vi "Camera Get connected Cameras.vi"() -> (1 "Product":string[](array[string]), 3 "Camera List":string[](array[string]))   [LabVIEW 2025]
uses:
  <vilib>/vision/driver/NI_Vision_Acquisition_Software.lvlib
panel:
  out "Camera Information Array 2":T1(array[cluster]) {"BusType" format="%x"; "SerialNumberLow" format="%.0x"; "SerialNumberHigh" format="%.0x"}
  out "Camera Information Array":T1(array[cluster]) {"BusType" format="%x"; "SerialNumberLow" format="%.0x"; "SerialNumberHigh" format="%.0x"}
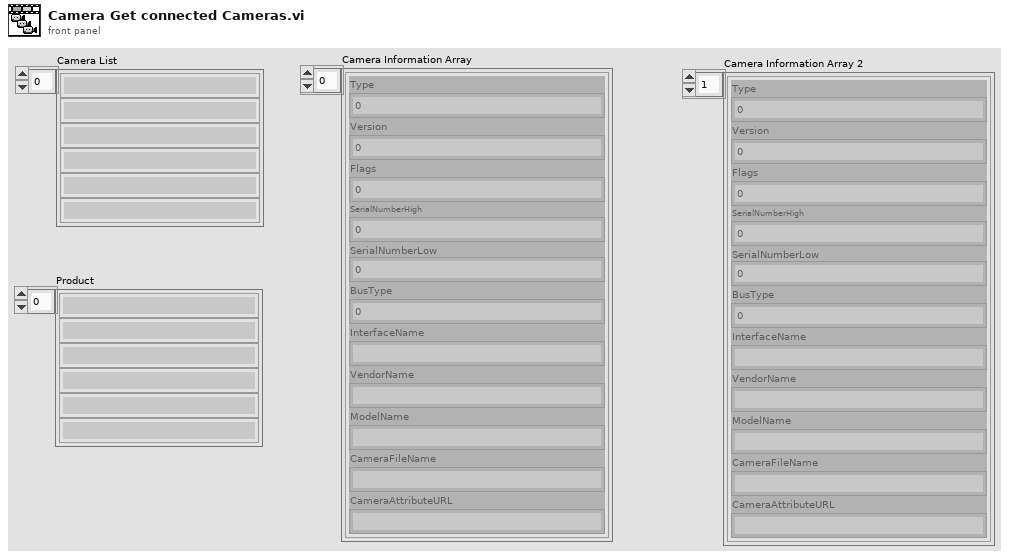
[diagram p1: front panel]
types:
  T1 = cluster{"Type":u32, "Version":u32, "Flags":u32, "SerialNumberHigh":u32, "SerialNumberLow":u32, "BusType":u32, "InterfaceName":string, "VendorName":string, "ModelName":string, "CameraFileName":string, "CameraAttributeURL":string}[]
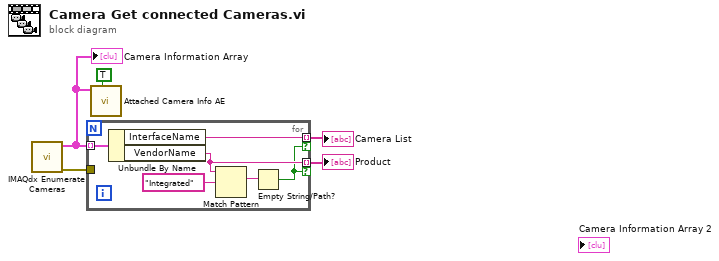
[diagram p0: block diagram]
diagram:
  n1 = call <vilib>:"IMAQdx Enumerate Cameras.vi"() -> ("error out"=w4:errorcluster, "Camera Information Array"=w3:T1)  [unwired: 10 in]
  "Camera Information Array" <- w3
  n2 = for {
    tunnel: w3 -> [w11] mode=indexing
    tunnel: [w10] -> w2 mode=indexing if=w6
    tunnel: [w8] -> w5 mode=indexing if=w6
    tunnel: w4 -> [_]
    n3 = Unbundle By Name(w11) -> ("InterfaceName"=w10:string, "VendorName"=w8:string)
    n4 = Match Pattern(string=w8, regular expression="Integrated") -> (match substring=w7:string)  [unwired: 1 in, 3 out]
    n5 = Empty String/Path?(string/path=w7) -> (empty?=w6:bool)
  }
  "Camera List" <- w2
  "Product" <- w5
  n6 = call "Attached Camera Info AE.vi"("update"=TRUE, "Camera Information Array"=w3) -> ()  [unwired: 9 in, 1 out]
